vi "Convert with Linear Calibration (2D, XY Point).vi"(10 "Linear Calibration 2D":T1, 11 "A":T2) -> (3 "A*":T2)   [LabVIEW 2011, in "COSYLib.lvlib"]
doc: "Calculates Y=AX+B, with A and B taken from a <B>Linear Calibration</B> cluster."
uses:
  COSYLib.lvlib
  XY Point.ctl
  Linear Calibration 2D.ctl
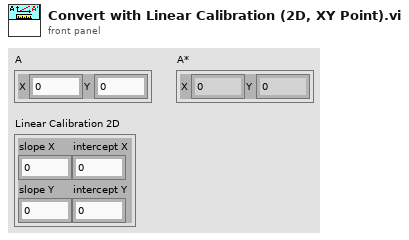
[diagram p1: front panel]
types:
  T1 = typedef "COSYLib.lvlib/Linear Calibration 2D.ctl" = cluster{"slope X":dbl, "intercept X":dbl, "slope Y":dbl, "intercept Y":dbl}
  T2 = typedef "COSYLib.lvlib/XY Point.ctl" = cluster{"X":dbl, "Y":dbl}
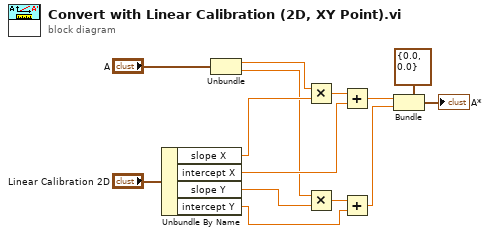
[diagram p0: block diagram]
diagram:
  n1 = Unbundle By Name("Linear Calibration 2D") -> ("slope X"=w10:dbl, "intercept X"=w9:dbl, "slope Y"=w7:dbl, "intercept Y"=w6:dbl)
  n2 = Unbundle("A") -> ("X"=w8:dbl, "Y"=w5:dbl)
  n3 = Multiply(x=w8, y=w10) -> (x*y=w14:dbl)
  n4 = Multiply(x=w5, y=w7) -> (x*y=w12:dbl)
  n5 = Add(x=w14, y=w9) -> (x+y=w4:dbl)
  n6 = Add(x=w12, y=w6) -> (x+y=w3:dbl)
  n7 = Bundle(cluster=T2 {"X"=0.0, "Y"=0.0} ("A"), "X"=w4, "Y"=w3) -> (→"A*":T2)
